vi "movePI.vi"(2 "PI Stage Error":errorcluster, 3 "move to position":dbl=0.00015 format="%.5f") -> (0 "final position":dbl, 1 "PI Stage Error 2":errorcluster)   [LabVIEW 2014]
panel:
  out "Position":dbl[](array[numeric]) format="%.6f"
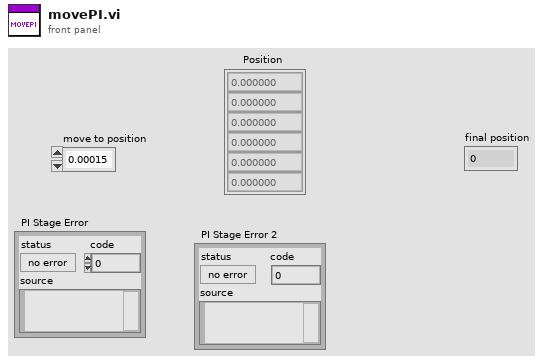
[diagram p1: front panel]
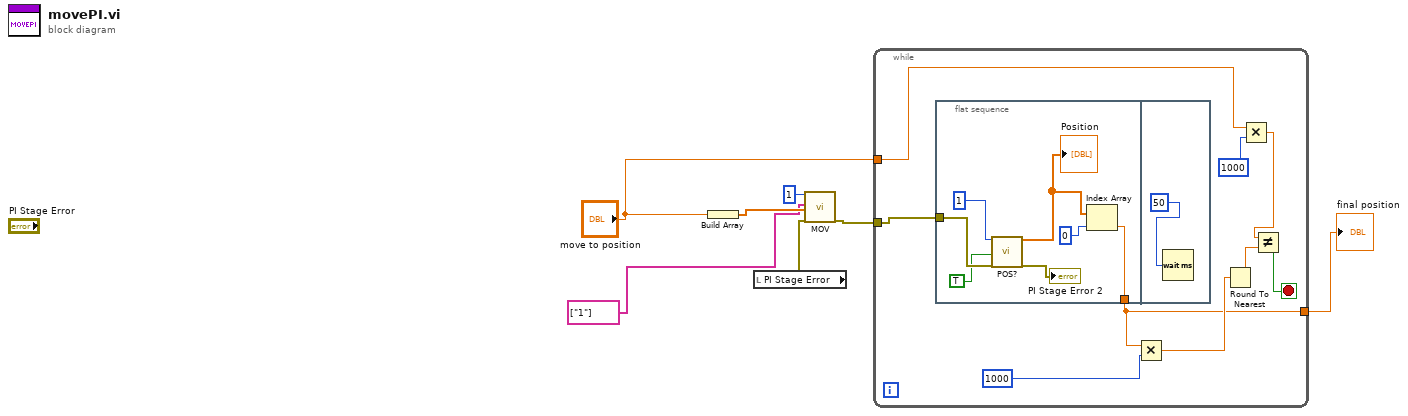
[diagram p0: block diagram]
diagram:
  n1 = Build Array("move to position") -> (w7:dbl[])
  n2 = local read "PI Stage Error"() -> (w6:errorcluster)
  n3 = call "MOV.vi"("System no."=1, "Axes to move"=string[] ["1"] ("Conn. Axes"), "Position values"=w7, "error in"=w6) -> ("error out"=w3:errorcluster)  [unwired: 15 in]
  n4 = while {
    tunnel: "move to position" -> [w13]
    tunnel: w3 -> [w15]
    tunnel: [w8] -> w1
    stop <- w16 stop-if-true
    n5 = flat-sequence {
      tunnel: w15 -> [w23]
      tunnel: [w17] -> w8
      frame #0 {
        n6 = call "POS?.vi"("System no."=1, "All axes?"=TRUE, "error in"=w23) -> ("Position"=w19:dbl[], "error out"=→"PI Stage Error 2":errorcluster)  [unwired: 15 in]
        "Position" <- w19
        n7 = Index Array(array=w19, index=0) -> (element=w17:dbl)
      }
      frame #1 {
        n8 = Wait (ms)(milliseconds to wait=50) -> ()  [unwired: 1 out]
      }
    }
    n9 = Multiply(x=w8, y=1000 ("System no.")) -> (x*y=w9:dbl)
    n10 = Round To Nearest(number=w9) -> (nearest integer value=w14:dbl)
    n11 = Multiply(x=w13, y=1000 ("System no.")) -> (x*y=w11:dbl)
    n12 = Not Equal?(x=w11, y=w14) -> (x != y?=w16:bool)
  }
  "final position" <- w1
